vi "Insert Element.vi"(8 "error in (no error)":errorcluster, 10 "Element":u32, 11 "Ordered Array in":refnum<class "Ordered Array.lvclass">) -> (0 "error out":errorcluster, 3 "Ordered Array out":refnum<class "Ordered Array.lvclass">)   [LabVIEW 2019, in "Ordered Array.lvclass"]
uses:
  Ordered Array.lvclass
  Ordered Array.lvclass/Ordered Array.ctl
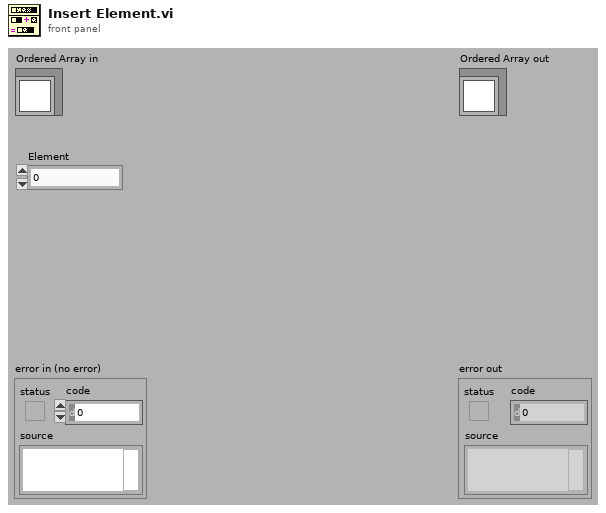
[diagram p1: front panel]
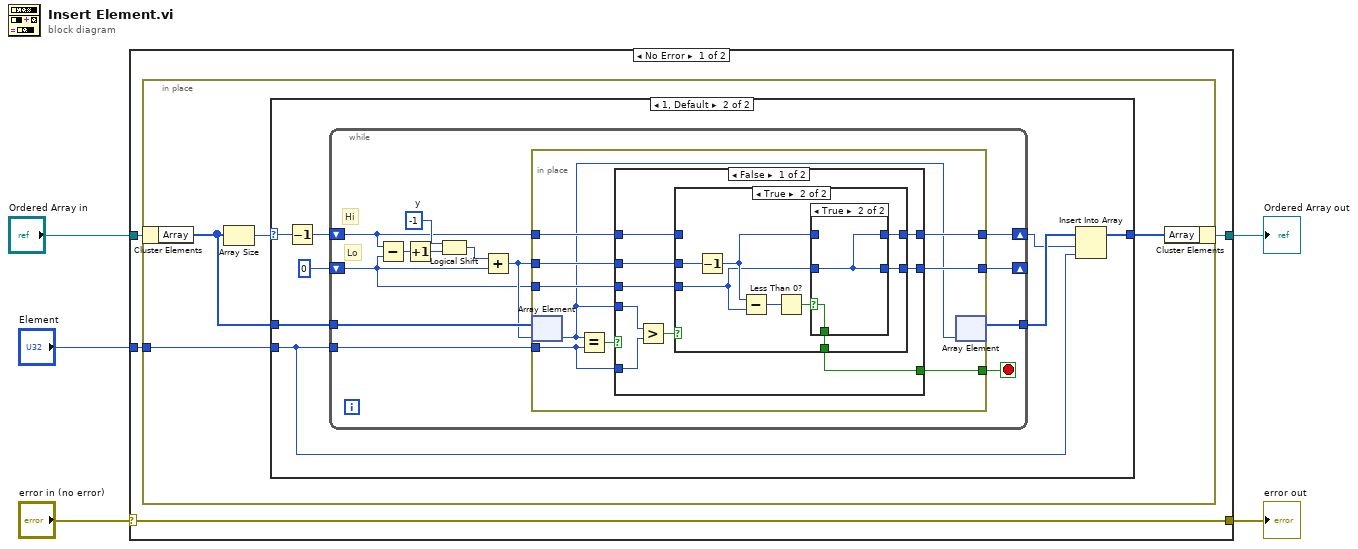
[diagram p0: block diagram]
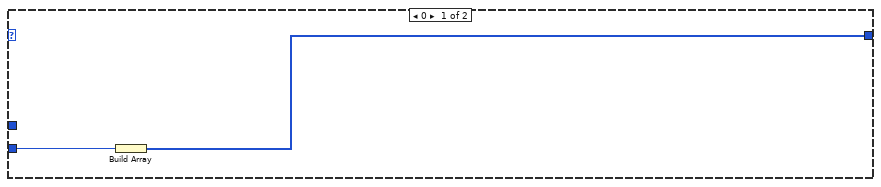
[diagram p2: hidden frame]
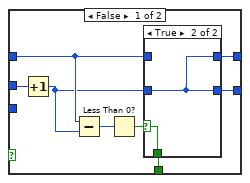
[diagram p3: hidden frame]
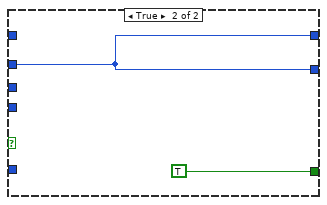
[diagram p6: hidden frame]
diagram:
  n1 = case shown="No Error" "error in (no error)" {
    selector: "error in (no error)" -> [w6 w84]
    tunnel: [w6 w84] -> w4
    tunnel: [w7 w83] -> w2
    tunnel: "Ordered Array in" -> [w9 w83]
    tunnel: "Element" -> [w8 _]
    frame No Error {
      n2 = in-place {
        in-place-border: w8 -> [w12]
        n3 = in-place-cluster #1(w9) -> ("Array"=w10:u32[])
        n4 = Array Size(array=w10) -> (size(s)=w13:i32)
        n5 = case shown="1, Default" w13 {
          selector: w13 -> [_ w22]
          tunnel: w12 -> [w15 w20]
          tunnel: [w14 w21] -> w11
          tunnel: w10 -> [_ w19]
          frame 0 {
            n6 = Build Array(w15) -> (w14:u32[])
          }
          frame 1, Default {
            n7 = Decrement(x=w22) -> (x-1=w17:i32)
            n8 = while {
              shift-right: [w27] -> _
              shift-left: 0 ("Lo") -> [w30]
              shift-right: [w28] -> w16
              shift-left: w17 -> [w29]
              tunnel: w19 -> [w33]
              tunnel: w20 -> [w32]
              tunnel: [w26] -> w18
              stop <- w24 stop-if-true
              w35 = i8 -1  # y
              # "Lo"
              # "Hi"
              n9 = Subtract(x=w29, y=w30) -> (x-y=w36:i32)
              n10 = Increment(x=w36) -> (x+1=w25:i32)
              n11 = Logical Shift(y=w35, x=w25) -> (x << y=w34:i32)
              n12 = Add(x=w34, y=w30) -> (x+y=w31:i32)
              n13 = in-place {
                in-place-border: w32 -> [w44]
                in-place-border: [w43] -> w28
                in-place-border: w31 -> [w42]
                in-place-border: [w41] -> w27
                in-place-border: w30 -> [w40]
                in-place-border: w29 -> [w39]
                in-place-border: [w37] -> w24
                n14 = in-place-array #2(w33, w31) -> (w38:u32)
                n15 = Equal?(x=w38, y=w44) -> (x = y?=w45:bool)
                n16 = case shown="False" w45 {
                  tunnel: w38 -> [w54 _]
                  tunnel: w44 -> [w53 _]
                  tunnel: [w51 w82] -> w43
                  tunnel: w42 -> [w50 w82]
                  tunnel: [w49 w82] -> w41
                  tunnel: w40 -> [w48 _]
                  tunnel: w39 -> [w47 _]
                  tunnel: [w46 TRUE] -> w37
                  frame False {
                    n17 = Greater?(x=w54, y=w53) -> (0:w52:bool)
                    n18 = case shown="True" w52 {
                      tunnel: [w59 w71] -> w51
                      tunnel: w50 -> [w62 w75]
                      tunnel: [w58 w72] -> w49
                      tunnel: w48 -> [_ w68]
                      tunnel: w47 -> [w57 _]
                      tunnel: [w55 w69] -> w46
                      frame False {
                        n19 = Increment(x=w62) -> (x+1=w56:i32)
                        n20 = Subtract(x=w57, y=w56) -> (x-y=w60:i32)
                        n21 = Less Than 0?(x=w60) -> (x < 0?=w61:bool)
                        n22 = case shown="True" w61 {
                          selector: w61 -> [w63 w67]
                          tunnel: [w65 w66] -> w58
                          tunnel: w56 -> [w65 w66]
                          tunnel: [w64 w66] -> w59
                          tunnel: w57 -> [w64 _]
                          tunnel: [w63 w67] -> w55
                          frame False {
                          }
                          frame True {
                          }
                        }
                      }
                      frame True {
                        n23 = Decrement(x=w75) -> (x-1=w70:i32)
                        n24 = Subtract(x=w70, y=w68) -> (x-y=w74:i32)
                        n25 = Less Than 0?(x=w74) -> (x < 0?=w73:bool)
                        n26 = case shown="True" w73 {
                          selector: w73 -> [w76 w80]
                          tunnel: [w78 w79] -> w72
                          tunnel: w68 -> [w78 w79]
                          tunnel: [w77 w79] -> w71
                          tunnel: w70 -> [w77 _]
                          tunnel: [w76 w80] -> w69
                          frame False {
                          }
                          frame True {
                          }
                        }
                      }
                    }
                  }
                  frame True {
                  }
                }
                n27 = in-place-array #2(w38) -> (w26:u32[])  [unwired: 1 out]
              }
            }
            n28 = Insert Into Array(array=w18, index=w16, new element=w20) -> (w21:u32[])
          }
        }
        n29 = in-place-cluster #1("Array"=w11) -> (w7:refnum<class "Ordered Array.lvclass">)
      }
    }
    frame Error {
    }
  }
  "error out" <- w4
  "Ordered Array out" <- w2
